vi "RevolverOcelotMkII.vi"(8 "Triggers":dbl(knob) scale=-1.0..1.0, 9 "RCW (X2)":dbl(slide) scale=-1.0..1.0, 10 "FWD (Y)":dbl(slide) scale=-1.0..1.0, 11 "STR (X)":dbl(slide) scale=-1.0..1.0) -> (0 "FRD":dbl(slide) scale=-1.0..1.0, 1 "FLD":dbl(slide) scale=-1.0..1.0, 2 "BRS":dbl(knob) scale=0.0..360.0, 3 "BLS":dbl(knob) scale=0.0..360.0, 4 "BLD":dbl(slide) scale=-1.0..1.0, 5 "FRS":dbl(knob) scale=0.0..360.0, 6 "BRD":dbl(slide) scale=-1.0..1.0, 7 "FLS":dbl(knob) scale=0.0..360.0)   [LabVIEW 2012]
uses:
  <vilib>/Rock Robotics/WPI/DriverStation/DriverStationLCD/WPI_DriverStationLCDLCDLine.ctl
panel:
  # "If going left, spin right\n\nIf going right, spin left"
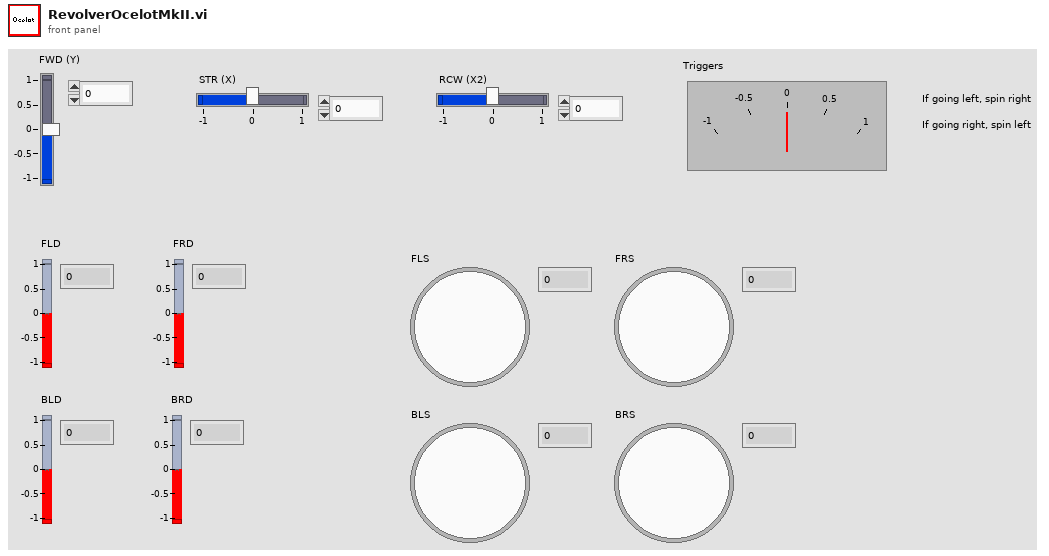
[diagram p1: front panel]
types:
  T1 = typedef "WPI_DriverStationLCDLCDLine.ctl" = enum16{"Main - Line 1", "User - Line 2", "User - Line 3", "User - Line 4", "User - Line 5", "User - Line 6"}
  T2 = cluster{"WD1":dbl, "WD2":dbl, "WD3":dbl, "WD4":dbl}
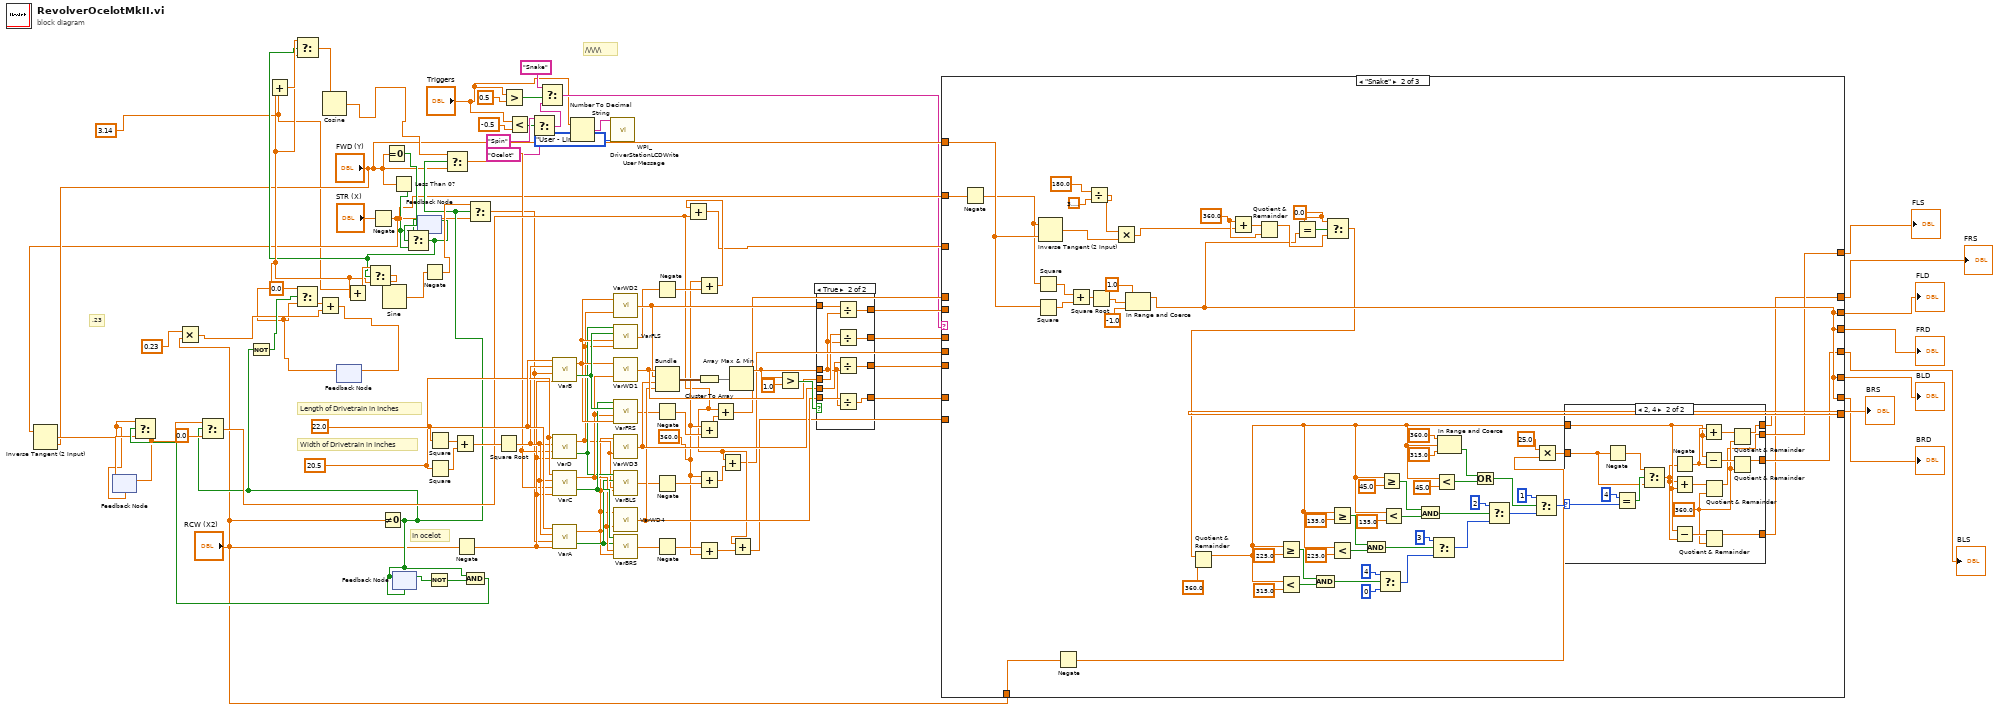
[diagram p0: block diagram]
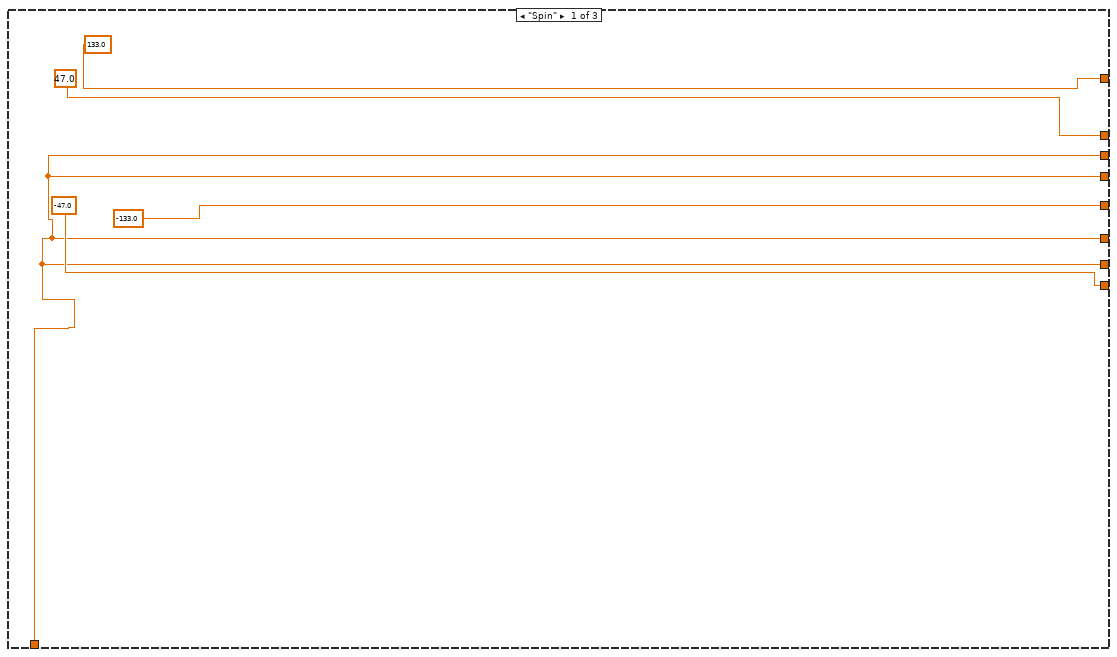
[diagram p2: hidden frame]
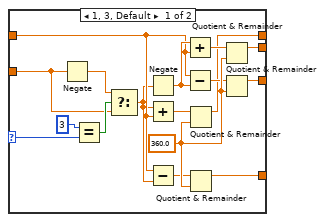
[diagram p3: hidden frame]
diagram:
  w1 = 3.14 ("x")
  w62 = 360.0
  w95 = 20.5 ("W")
  w96 = 22.0 ("L")
  # "/\\/\\/\\/\\"
  # ".23"
  # "In ocelot"
  # "Length of Drivetrain in Inches"
  # "Width of Drivetrain in Inches"
  n1 = Multiply(x=0.23, y="RCW (X2)") -> (x*y=w49:dbl)
  n2 = feedback #1() -> (w38:dbl)  [unwired: 1 in]
  n3 = Add(x=w38, y=w1) -> (x+y=w41:dbl)
  n4 = Add(x=w1, y=w38) -> (x+y=w39:dbl)
  n5 = Negate(x="STR (X)") -> (-x=w15:dbl)
  n6 = Inverse Tangent (2 Input)(1:"FWD (Y)", 2:w15) -> (0:w54:dbl)
  n7 = feedback #2(w54) -> (w56:dbl)
  n8 = Not Equal To 0?(x="RCW (X2)") -> (x != 0?=w48:bool)
  n9 = Not(x=w48) -> (.not. x?=w64:bool)
  n10 = Select(t=0.0, s=w64, f=w38) -> (s? t:f=w66:dbl)
  n11 = Add(x=w66, y=w49) -> (x+y=w45:dbl)
  n12 = feedback-in #1(w45) -> ()
  n13 = Equal To 0?(x="FWD (Y)") -> (x = 0?=w37:bool)
  n14 = Less Than 0?(x="FWD (Y)") -> (x < 0?=w35:bool)
  n15 = feedback-in #3(w48) -> ()
  n16 = feedback #3(w48) -> (w61:bool)
  n17 = feedback #4(w35) -> (w36:bool)
  n18 = Select(t=w36, s=w37, f=w35) -> (s? t:f=w34:bool)
  n19 = Select(t=w41, s=w34, f=w38) -> (s? t:f=w42:dbl)
  n20 = Cosine(x=w42) -> (cos(x)=w43:dbl)
  n21 = Select(t=w39, s=w34, f=w38) -> (s? t:f=w40:dbl)
  n22 = Sine(x=w40) -> (sin(x)=w44:dbl)
  n23 = feedback-in #4(w34) -> ()
  n24 = Negate(x=w44) -> (-x=w63:dbl)
  n25 = Not(x=w61) -> (.not. x?=w60:bool)
  n26 = Square(x=w96) -> (x^2=w99:dbl)
  n27 = Square(x=w95) -> (x^2=w98:dbl)
  n28 = Select(t=w43, s=w48, f="FWD (Y)") -> (s? t:f=w47:dbl)
  n29 = Add(x=w99, y=w98) -> (x+y=w97:dbl)
  n30 = Negate(x="RCW (X2)") -> (-x=w67:dbl)
  n31 = And(x=w48, y=w60) -> (x .and. y?=w57:bool)
  n32 = Select(t=w54, s=w57, f=w56) -> (s? t:f=w55:dbl)
  n33 = feedback-in #2(w55) -> ()
  n34 = Select(t=w55, s=w48, f=0.0) -> (s? t:f=w50:dbl)
  n35 = Select(t=w63, s=w48, f=w15) -> (s? t:f=w46:dbl)
  n36 = Square Root(x=w97) -> (sqrt(x)=w94:dbl)
  n37 = Greater?(x="Triggers", y=0.5) -> (0:w14:bool)
  n38 = Less?(x="Triggers", y=-0.5 ("x")) -> (x < y?=w11:bool)
  n39 = Select(t="Spin", s=w11, f="Ocelot") -> (s? t:f=w10:string)
  n40 = Select(t="Snake", s=w14, f=w10) -> (s? t:f=w8:string)
  n41 = call "VarB.vi"("RCW (X2)"=w67, "STR (X)"=w46, "R"=w94, "L"=w96) -> ("B = 0?"=w84:bool, "B"=w83:dbl)
  n42 = call "VarD.vi"("RCW (X2)"=w67, "FWD (Y)"=w47, "R"=w94, "W"=w95) -> ("x = 0?"=w80:bool, "D"=w78:dbl)
  n43 = call "VarC.vi"("RCW (X2)"=w67, "FWD (Y)"=w47, "R"=w94, "W"=w95) -> ("C = 0?"=w82:bool, "C"=w81:dbl)
  n44 = call "VarA.vi"("RCW (X2)"=w67, "STR (X)"=w46, "R"=w94, "L"=w96) -> ("A = 0?"=w79:bool, "A"=w77:dbl)
  n45 = Number To Decimal String(number="Triggers") -> (decimal integer string=w7:string)  [unwired: 1 in]
  n46 = call <vilib>:"WPI_DriverStationLCDWrite User Message.vi"("line text"=w7, "line"=WPI_DriverStationLCDLCDLine."User - Line 2") -> ()  [unwired: 13 in, 1 out]
  n47 = call "VarWD2.vi"("D"=w78, "B"=w83) -> ("WD2"=w88:dbl)
  n48 = call "VarFLS.vi"("D"=w78, "B"=w83, "B=0"=w84, "D=0"=w80) -> ("FLS"=w68:dbl)
  n49 = call "VarWD1.vi"("C"=w81, "B"=w83) -> ("WD1"=w89:dbl)
  n50 = call "VarFRS.vi"("B"=w83, "C"=w81, "B=0"=w84, "C=0"=w82) -> ("FRS"=w69:dbl)
  n51 = call "VarWD3.vi"("D"=w78, "A"=w77) -> ("WD3"=w87:dbl)
  n52 = call "VarBLS.vi"("A"=w77, "D"=w78, "A=0"=w79, "D=0"=w80) -> ("BLS"=w70:dbl)
  n53 = call "VarWD4.vi"("C"=w81, "A"=w77) -> ("WD4"=w86:dbl)
  n54 = call "VarBRS.vi"("A"=w77, "C"=w81, "A=0"=w79, "C=0"=w82) -> ("BRS"=w72:dbl)
  n55 = Negate(x=w68) -> (-x=w76:dbl)
  n56 = Negate(x=w69) -> (-x=w75:dbl)
  n57 = Negate(x=w70) -> (-x=w74:dbl)
  n58 = Negate(x=w72) -> (-x=w73:dbl)
  n59 = Bundle("WD1"=w89, "WD2"=w88, "WD3"=w87, "WD4"=w86) -> (w92:T2)  [unwired: 1 in]
  n60 = Add(x=w62, y=w76) -> (x+y=w53:dbl)
  n61 = Add(x=w53, y=w50) -> (x+y=w32:dbl)
  n62 = Cluster To Array(cluster=w92) -> (array=w93:dbl[])
  n63 = Add(x=w62, y=w75) -> (x+y=w52:dbl)
  n64 = Add(x=w62, y=w74) -> (x+y=w51:dbl)
  n65 = Add(x=w73, y=w62) -> (x+y=w71:dbl)
  n66 = Add(x=w50, y=w52) -> (x+y=w30:dbl)
  n67 = Add(x=w50, y=w51) -> (x+y=w28:dbl)
  n68 = Array Max & Min(array=w93) -> (max value=w85:dbl)  [unwired: 3 out]
  n69 = Add(x=w50, y=w71) -> (x+y=w26:dbl)
  n70 = Greater?(x=w85, y=1.0) -> (0:w90:bool)
  n71 = case shown="True" w90 {
    tunnel: [w103 w108] -> w22
    tunnel: w89 -> [w103 w111]
    tunnel: w88 -> [w102 w112]
    tunnel: w87 -> [w101 w109]
    tunnel: w86 -> [w100 w110]
    tunnel: [w102 w107] -> w25
    tunnel: [w101 w106] -> w20
    tunnel: [w100 w104] -> w18
    tunnel: w85 -> [_ w105]
    frame False {
    }
    frame True {
      n72 = Divide(x=w112, y=w105) -> (x/y=w107:dbl)
      n73 = Divide(x=w111, y=w105) -> (x/y=w108:dbl)
      n74 = Divide(x=w109, y=w105) -> (x/y=w106:dbl)
      n75 = Divide(x=w110, y=w105) -> (x/y=w104:dbl)
    }
  }
  n76 = case shown="\"Snake\"" w8 {
    tunnel: [133.0 w124 w220] -> w33
    tunnel: w32 -> [_ _ w220]
    tunnel: [47.0 w122 w219] -> w31
    tunnel: w30 -> [_ _ w219]
    tunnel: [-133.0 w123 w218] -> w29
    tunnel: w28 -> [_ _ w218]
    tunnel: [-47.0 w125 w217] -> w27
    tunnel: w26 -> [_ _ w217]
    tunnel: w25 -> [_ _ w216]
    tunnel: [w113 w127 w216] -> w24
    tunnel: [w113 w127 w215] -> w23
    tunnel: w22 -> [_ _ w215]
    tunnel: [w113 w127 w214] -> w21
    tunnel: w20 -> [_ _ w214]
    tunnel: [w113 w127 w213] -> w19
    tunnel: w18 -> [_ _ w213]
    tunnel: "RCW (X2)" -> [w113 w121 _]
    tunnel: "FWD (Y)" -> [_ w129 _]
    tunnel: w15 -> [_ w128 _]
    frame "Spin" {
    }
    frame "Snake" {
      w130 = 0.0
      w137 = 360.0
      n77 = Negate(x=w128) -> (-x=w119:dbl)
      n78 = Square(x=w119) -> (x^2=w140:dbl)
      n79 = Square(x=w129) -> (x^2=w141:dbl)
      n80 = Inverse Tangent (2 Input)(1:w129, 2:w119) -> (0:w142:dbl)
      n81 = Negate(x=w121) -> (-x=w120:dbl)
      n82 = Add(x=w140, y=w141) -> (x+y=w139:dbl)
      n83 = Divide(x=180.0, y=3.141592653589793) -> (x/y=w143:dbl)
      n84 = Square Root(x=w139) -> (sqrt(x)=w133:dbl)
      n85 = Multiply(x=w143, y=w142) -> (x*y=w136:dbl)
      n86 = In Range and Coerce(upper limit=1.0, x=w133, lower limit=-1.0 ("upper limit")) -> (coerced(x)=w127:dbl)  [unwired: 1 out]
      n87 = Add(x=w137, y=w136) -> (x+y=w138:dbl)
      n88 = Quotient & Remainder(x=w138, y=w137) -> (x-y*floor(x/y)=w134:dbl)  [unwired: 1 out]
      n89 = Equal?(x=w130, y=w127) -> (x = y?=w135:bool)
      n90 = Select(t=w130, s=w135, f=w134) -> (s? t:f=w126:dbl)
      n91 = Quotient & Remainder(x=w126, y=360.0) -> (x-y*floor(x/y)=w146:dbl)  [unwired: 1 out]
      n92 = Greater Or Equal?(x=w146, y=225.0) -> (x >= y?=w161:bool)
      n93 = Less?(x=w146, y=315.0) -> (x < y?=w162:bool)
      n94 = And(x=w161, y=w162) -> (x .and. y?=w160:bool)
      n95 = Greater Or Equal?(x=w146, y=135.0) -> (x >= y?=w168:bool)
      n96 = Less?(x=w146, y=225.0) -> (x < y?=w167:bool)
      n97 = And(x=w168, y=w167) -> (x .and. y?=w154:bool)
      n98 = Select(t=4, s=w160, f=0) -> (s? t:f=w159:i32)
      n99 = Greater Or Equal?(x=w146, y=45.0) -> (x >= y?=w169:bool)
      n100 = Less?(x=w146, y=135.0) -> (x < y?=w170:bool)
      n101 = And(x=w169, y=w170) -> (x .and. y?=w155:bool)
      n102 = Select(t=3, s=w154, f=w159) -> (s? t:f=w158:i32)
      n103 = Less?(x=w146, y=45.0) -> (x < y?=w174:bool)
      n104 = In Range and Coerce(upper limit=360.0, x=w146, lower limit=315.0) -> (In Range?=w173:bool)  [unwired: 1 out]
      n105 = Or(x=w173, y=w174) -> (x .or. y?=w156:bool)
      n106 = Select(t=2, s=w155, f=w158) -> (s? t:f=w157:i32)
      n107 = Select(t=1, s=w156, f=w157) -> (s? t:f=w148:i32)
      n108 = Multiply(x=25.0, y=w120) -> (x*y=w178:dbl)
      n109 = case shown="2, 4" w148 {
        selector: w148 -> [w184 w200]
        tunnel: [w186 w206] -> w123
        tunnel: [w187 w205] -> w125
        tunnel: [w185 w204] -> w122
        tunnel: [w188 w203] -> w124
        tunnel: w146 -> [w189 w202]
        tunnel: w178 -> [w180 w197]
        frame 1, 3, Default {
          w195 = 360.0 ("y")
          n110 = Negate(x=w180) -> (-x=w181:dbl)
          n111 = Equal?(x=3, y=w184) -> (x = y?=w182:bool)
          n112 = Select(t=w181, s=w182, f=w180) -> (s? t:f=w179:dbl)
          n113 = Negate(x=w179) -> (-x=w190:dbl)
          n114 = Add(x=w179, y=w189) -> (x+y=w193:dbl)
          n115 = Subtract(x=w189, y=w179) -> (x-y=w194:dbl)
          n116 = Add(x=w190, y=w189) -> (x+y=w191:dbl)
          n117 = Subtract(x=w189, y=w190) -> (x-y=w192:dbl)
          n118 = Quotient & Remainder(x=w193, y=w195) -> (x-y*floor(x/y)=w187:dbl)  [unwired: 1 out]
          n119 = Quotient & Remainder(x=w194, y=w195) -> (x-y*floor(x/y)=w185:dbl)  [unwired: 1 out]
          n120 = Quotient & Remainder(x=w191, y=w195) -> (x-y*floor(x/y)=w188:dbl)  [unwired: 1 out]
          n121 = Quotient & Remainder(x=w192, y=w195) -> (x-y*floor(x/y)=w186:dbl)  [unwired: 1 out]
        }
        frame 2, 4 {
          w207 = 360.0 ("y")
          n122 = Negate(x=w197) -> (-x=w198:dbl)
          n123 = Equal?(x=4, y=w200) -> (x = y?=w199:bool)
          n124 = Select(t=w198, s=w199, f=w197) -> (s? t:f=w196:dbl)
          n125 = Negate(x=w196) -> (-x=w212:dbl)
          n126 = Add(x=w196, y=w202) -> (x+y=w209:dbl)
          n127 = Subtract(x=w202, y=w196) -> (x-y=w208:dbl)
          n128 = Add(x=w212, y=w202) -> (x+y=w211:dbl)
          n129 = Subtract(x=w202, y=w212) -> (x-y=w210:dbl)
          n130 = Quotient & Remainder(x=w209, y=w207) -> (x-y*floor(x/y)=w203:dbl)  [unwired: 1 out]
          n131 = Quotient & Remainder(x=w208, y=w207) -> (x-y*floor(x/y)=w204:dbl)  [unwired: 1 out]
          n132 = Quotient & Remainder(x=w211, y=w207) -> (x-y*floor(x/y)=w205:dbl)  [unwired: 1 out]
          n133 = Quotient & Remainder(x=w210, y=w207) -> (x-y*floor(x/y)=w206:dbl)  [unwired: 1 out]
        }
      }
    }
    frame "Ocelot", Default {
    }
  }
  "FRD" <- w23
  "FLD" <- w24
  "BLD" <- w21
  "BRD" <- w19
  "FLS" <- w33
  "FRS" <- w31
  "BRS" <- w27
  "BLS" <- w29
